vi "Set Property.vi"(0 "SLSC Remote in":refnum<class "SLSC Remote.lvclass">, 1 "property type":T1, 5 "resources":string="$DefaultDevices", 7 "property":refnum<k21>, 9 "property value":variant, 11 "error in (no error)":errorcluster) -> (4 "SLSC Remote out":refnum<class "SLSC Remote.lvclass">, 15 "error out":errorcluster)   [LabVIEW 2015, in "SLSC Remote.lvclass"]
uses:
  SLSC Remote.lvclass
  SLSC Interface Class/Property Type.ctl
  <vilib>/NI/i3 JSON/JSON Generation/Create Value Files/Create Value - Object.vi
  <vilib>/NI/i3 JSON/JSON Generation/Add Object Parameter Files/Add Object Parameter - String.vi
  <vilib>/NI/i3 JSON/JSON Generation/Add Object Parameter Files/Add Object Parameter - Numeric.vi
  <vilib>/NI/i3 JSON/JSON Generation/Add Object Parameter Files/Add Object Parameter - 1D Array Boolean.vi
  <vilib>/NI/i3 JSON/JSON Generation/Add Object Parameter Files/Add Object Parameter - 1D Array Double.vi
  <vilib>/NI/i3 JSON/JSON Generation/Add Object Parameter Files/Add Object Parameter - 1D Array String.vi
  <vilib>/NI/i3 JSON/JSON Generation/Add Object Parameter Files/Add Object Parameter - Boolean.vi
  <vilib>/NI/NI JSONRPC Server Framework/Classes/Server/Format Client Request (Auto-Increment).vi
  <vilib>/httpClient/POSTBuffer.vi
  <vilib>/NI/NI JSONRPC Server Framework/Classes/Server/JSONRPC Server.lvclass
  <vilib>/NI/i3 JSON/i3-json.lvlib
  <vilib>/httpClient/LabVIEWHTTPClient.lvlib
  SLSC Interface Class/SLSC Interface.lvclass
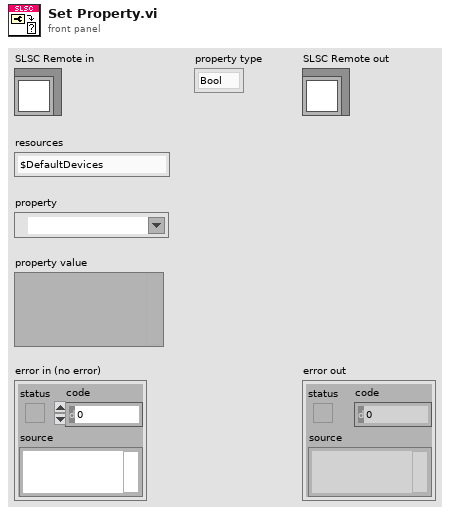
[diagram p1: front panel]
types:
  T1 = typedef "SLSC Interface.lvclass/Property Type.ctl" = enum16{"Bool", "DBL", "I32", "I64", "String", "U32", "U64", "1D Bool", "1D DBL", "1D I32", "1D I64", "1D String", "1D U32", "1D U64"}
  T2 = typedef "LabVIEWHTTPClient.lvlib/ClientHandle.ctl" = refnum<k1>
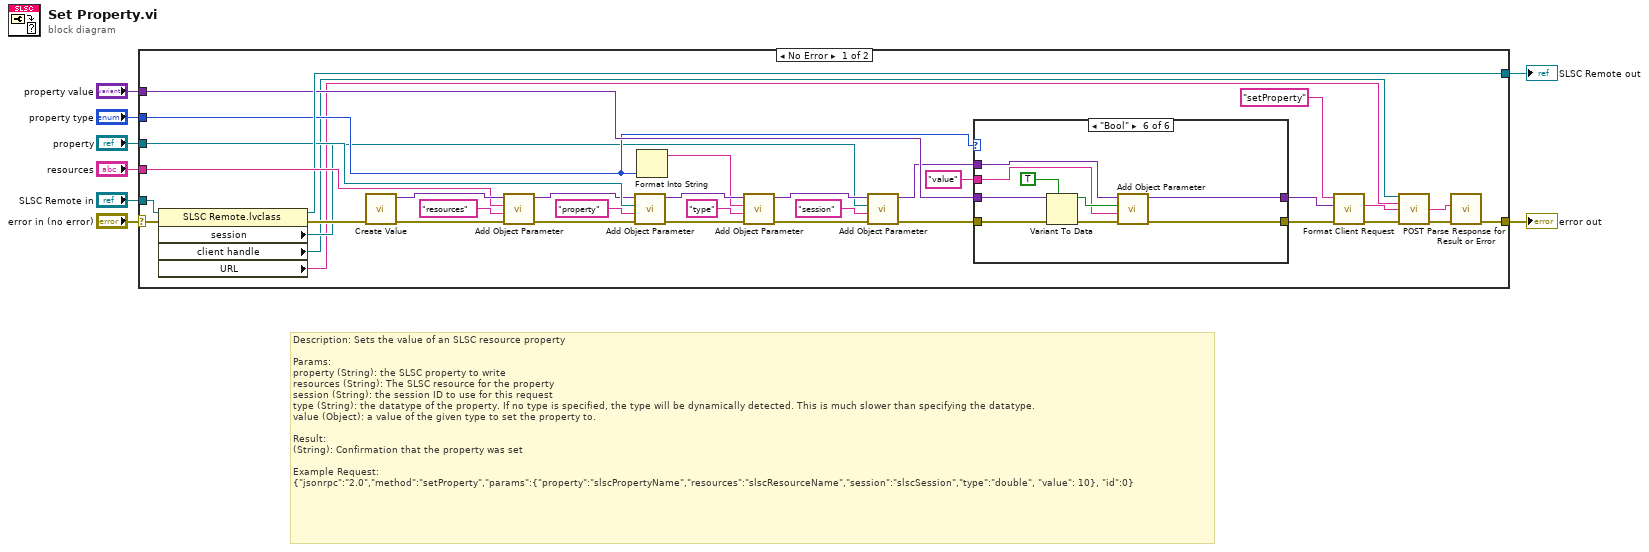
[diagram p0: block diagram]
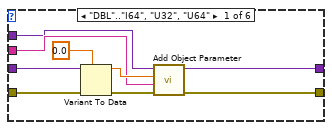
[diagram p2: hidden frame]
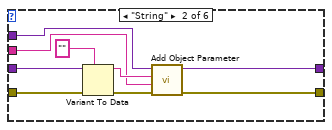
[diagram p3: hidden frame]
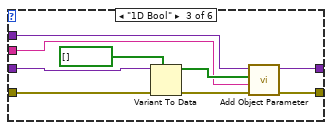
[diagram p4: hidden frame]
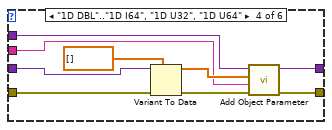
[diagram p5: hidden frame]
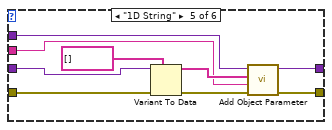
[diagram p6: hidden frame]
diagram:
  # "Description: Sets the value of an SLSC resource property\n\nParams:\nproperty (String): the SLSC property to write\nresources (String): The SLSC resource for the property\nsession (String): the session ID to use for this request\ntype (String): the datatype of the property. If no type is specified, the type will be dynamically detected. This is much slower than specifying the datatype.\nvalue (Object): a value of the given type to set the property to.\n\nResult:\n(String): Confirmation that the property was set\n\nExample Request: \n{\"jsonrpc\":\"2.0\",\"method\":\"setProperty\",\"params\":{\"property\":\"slscPropertyName\",\"resources\":\"slscResourceName\",\"session\":\"slscSession\",\"type\":\"double\", \"value\": 10}, \"id\":0}"
  n1 = case shown="No Error" "error in (no error)" {
    selector: "error in (no error)" -> [w34 w98]
    tunnel: "resources" -> [w42 _]
    tunnel: "SLSC Remote in" -> [w40 w99]
    tunnel: [w39 w99] -> w6
    tunnel: "property" -> [w37 _]
    tunnel: "property value" -> [w36 _]
    tunnel: "property type" -> [w30 _]
    tunnel: [w9 w98] -> w1
    frame No Error {
      n2 = property class="SLSC Remote.lvclass"(reference=w40, error in=w34) -> (reference out=w39:refnum<class "SLSC Remote.lvclass">, error out=w33:errorcluster, "session"=w22:refnum<k21>, "client handle"=w16:T2, "URL"=w15:string)
      n3 = call-poly <vilib>:"Create Value.vi"("error in (no error)"=w33) -> ("error out"=w32:errorcluster, "JSON Tree"=w43:variant)  [unwired: 9 in]
      n4 = call-poly <vilib>:"Add Object Parameter.vi"("error in (no error)"=w32, "Name"="resources", "String"=w42, "JSON Tree in (JSON Object)"=w43) -> ("error out"=w31:errorcluster, "JSON Tree out (JSON Object)"=w27:variant)  [unwired: 6 in]
      n5 = call-poly <vilib>:"Add Object Parameter.vi"("error in (no error)"=w31, "Name"="property", "String"=w37, "JSON Tree in (JSON Object)"=w27) -> ("error out"=w25:errorcluster, "JSON Tree out (JSON Object)"=w26:variant)  [unwired: 6 in]
      n6 = Format Into String(w30) -> (resulting string=w12:string)  [unwired: 3 in, 1 out]
      n7 = call-poly <vilib>:"Add Object Parameter.vi"("error in (no error)"=w25, "Name"="type" ("String"), "String"=w12, "JSON Tree in (JSON Object)"=w26) -> ("error out"=w23:errorcluster, "JSON Tree out (JSON Object)"=w24:variant)  [unwired: 6 in]
      n8 = call-poly <vilib>:"Add Object Parameter.vi"("error in (no error)"=w23, "Name"="session", "String"=w22, "JSON Tree in (JSON Object)"=w24) -> ("error out"=w19:errorcluster, "JSON Tree out (JSON Object)"=w20:variant)  [unwired: 6 in]
      n9 = case shown="\"Bool\"" w30 {
        tunnel: w36 -> [w52 w61 w70 w79 w88 w97]
        tunnel: "value" ("Name") -> [w49 w58 w67 w76 w85 w94]
        tunnel: w19 -> [w48 w57 w66 w75 w84 w93]
        tunnel: [w46 w55 w64 w73 w82 w91] -> w17
        tunnel: [w45 w54 w63 w72 w81 w90] -> w18
        tunnel: w20 -> [w44 w53 w62 w71 w80 w89]
        frame "DBL".."I64", "U32", "U64" {
          n10 = Variant To Data(error in=w48, type=0.0 ("Numeric"), Variant=w52) -> (data=w50:dbl, error out=w47:errorcluster)
          n11 = call-poly <vilib>:"Add Object Parameter.vi"("error in (no error)"=w47, "Name"=w49, "Numeric"=w50, "JSON Tree in (JSON Object)"=w44) -> ("error out"=w45:errorcluster, "JSON Tree out (JSON Object)"=w46:variant)  [unwired: 6 in]
        }
        frame "String" {
          n12 = Variant To Data(error in=w57, type="" ("Numeric"), Variant=w61) -> (data=w59:string, error out=w56:errorcluster)
          n13 = call-poly <vilib>:"Add Object Parameter.vi"("error in (no error)"=w56, "Name"=w58, "String"=w59, "JSON Tree in (JSON Object)"=w53) -> ("error out"=w54:errorcluster, "JSON Tree out (JSON Object)"=w55:variant)  [unwired: 6 in]
        }
        frame "1D Bool" {
          n14 = Variant To Data(error in=w66, type=bool[] [], Variant=w70) -> (data=w68:bool[], error out=w65:errorcluster)
          n15 = call-poly <vilib>:"Add Object Parameter.vi"("error in (no error)"=w65, "Name"=w67, "1D Boolean"=w68, "JSON Tree in (JSON Object)"=w62) -> ("error out"=w63:errorcluster, "JSON Tree out (JSON Object)"=w64:variant)  [unwired: 6 in]
        }
        frame "1D DBL".."1D I64", "1D U32", "1D U64" {
          n16 = Variant To Data(error in=w75, type=dbl[] [], Variant=w79) -> (data=w77:dbl[], error out=w74:errorcluster)
          n17 = call-poly <vilib>:"Add Object Parameter.vi"("error in (no error)"=w74, "Name"=w76, "1D Double"=w77, "JSON Tree in (JSON Object)"=w71) -> ("error out"=w72:errorcluster, "JSON Tree out (JSON Object)"=w73:variant)  [unwired: 6 in]
        }
        frame "1D String" {
          n18 = Variant To Data(error in=w84, type=string[] [], Variant=w88) -> (data=w86:string[], error out=w83:errorcluster)
          n19 = call-poly <vilib>:"Add Object Parameter.vi"("error in (no error)"=w83, "Name"=w85, "1D String"=w86, "JSON Tree in (JSON Object)"=w80) -> ("error out"=w81:errorcluster, "JSON Tree out (JSON Object)"=w82:variant)  [unwired: 6 in]
        }
        frame "Bool" {
          n20 = Variant To Data(error in=w93, type=TRUE, Variant=w97) -> (data=w95:bool, error out=w92:errorcluster)
          n21 = call-poly <vilib>:"Add Object Parameter.vi"("error in (no error)"=w92, "Name"=w94, "Boolean"=w95, "JSON Tree in (JSON Object)"=w89) -> ("error out"=w90:errorcluster, "JSON Tree out (JSON Object)"=w91:variant)  [unwired: 6 in]
        }
      }
      n22 = call-poly <vilib>:"Format Client Request.vi"("error in (no error)"=w18, "params"=w17, "method"="setProperty") -> ("error out"=w14:errorcluster, "Request String"=w28:string)  [unwired: 7 in]
      n23 = call-poly <vilib>:"POST.vi"("client handle"=w16, "url"=w15, "buffer"=w28, "error in (no error)"=w14) -> ("body"=w11:string, "error out"=w10:errorcluster)  [unwired: 8 in, 2 out]
      n24 = call <vilib>:"Parse Response for Result or Error.vi"("error in"=w10, "Response String In"=w11) -> ("error out"=w9:errorcluster)  [unwired: 7 in, 2 out]
    }
    frame Error {
    }
  }
  "error out" <- w1
  "SLSC Remote out" <- w6
